vi "Volts to Codes.vi"(9 "Number of Bits":i16=8, 10 "range (Vpp)":dbl=2.0, 11 "Data In":dbl) -> (3 "Data Out":i16)   [LabVIEW 2017]
doc: "This VI converts the dersired trigger level from volts to raw ADC codes for use on the FPGA VI."
panel:
  # "This VI converts the dersired trigger level from volts to raw ADC codes for use on the FPGA VI."
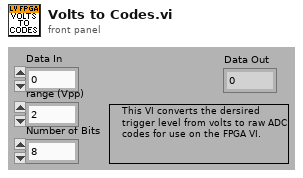
[diagram p1: front panel]
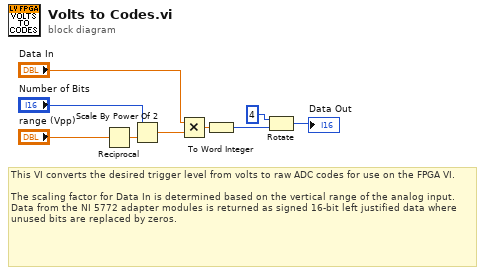
[diagram p0: block diagram]
diagram:
  # "This VI converts the desired trigger level from volts to raw ADC codes for use on the FPGA VI.  \n\nThe scaling factor for Data In is determined based on the vertical range of the analog input. Data from the NI 5772 adapter modules is returned as signed 16-bit left justified data where unused bits are replaced by zeros."
  n1 = Reciprocal(x="range (Vpp)") -> (1/x=w9:dbl)
  n2 = Scale By Power Of 2(n="Number of Bits", x=w9) -> (x*2^n=w5:dbl)
  n3 = Multiply(x="Data In", y=w5) -> (x*y=w7:dbl)
  n4 = To Word Integer(number=w7) -> (16bit integer=w6:i16)
  n5 = Rotate(1:w6, 2:i8 4 ("y")) -> (0:→"Data Out":i16)
